vi "WheelRotationsToFeet.vi"(4 "rotations":dbl) -> (1 "feet":dbl)   [LabVIEW 2019]
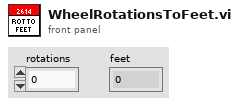
[diagram p1: front panel]
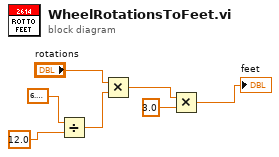
[diagram p0: block diagram]
diagram:
  n1 = Divide(x=6.283185307179586, y=12.0) -> (x/y=w4:dbl)
  n2 = Multiply(x="rotations", y=w4) -> (x*y=w3:dbl)
  n3 = Multiply(x=w3, y=3.0) -> (x*y=→"feet":dbl)
